vi "pattern_recogn+matching decay.vi"(10 "Image Out":T1, 11 "Path 3":path) -> (1 "Image":T1(plugin-control), 2 "x-y":i32, 3 "Matches (pixel)":T2(array[cluster]))   [LabVIEW 2015]
uses:
  <vilib>/vision/Image Controls.llb/IMAQ Image.ctl
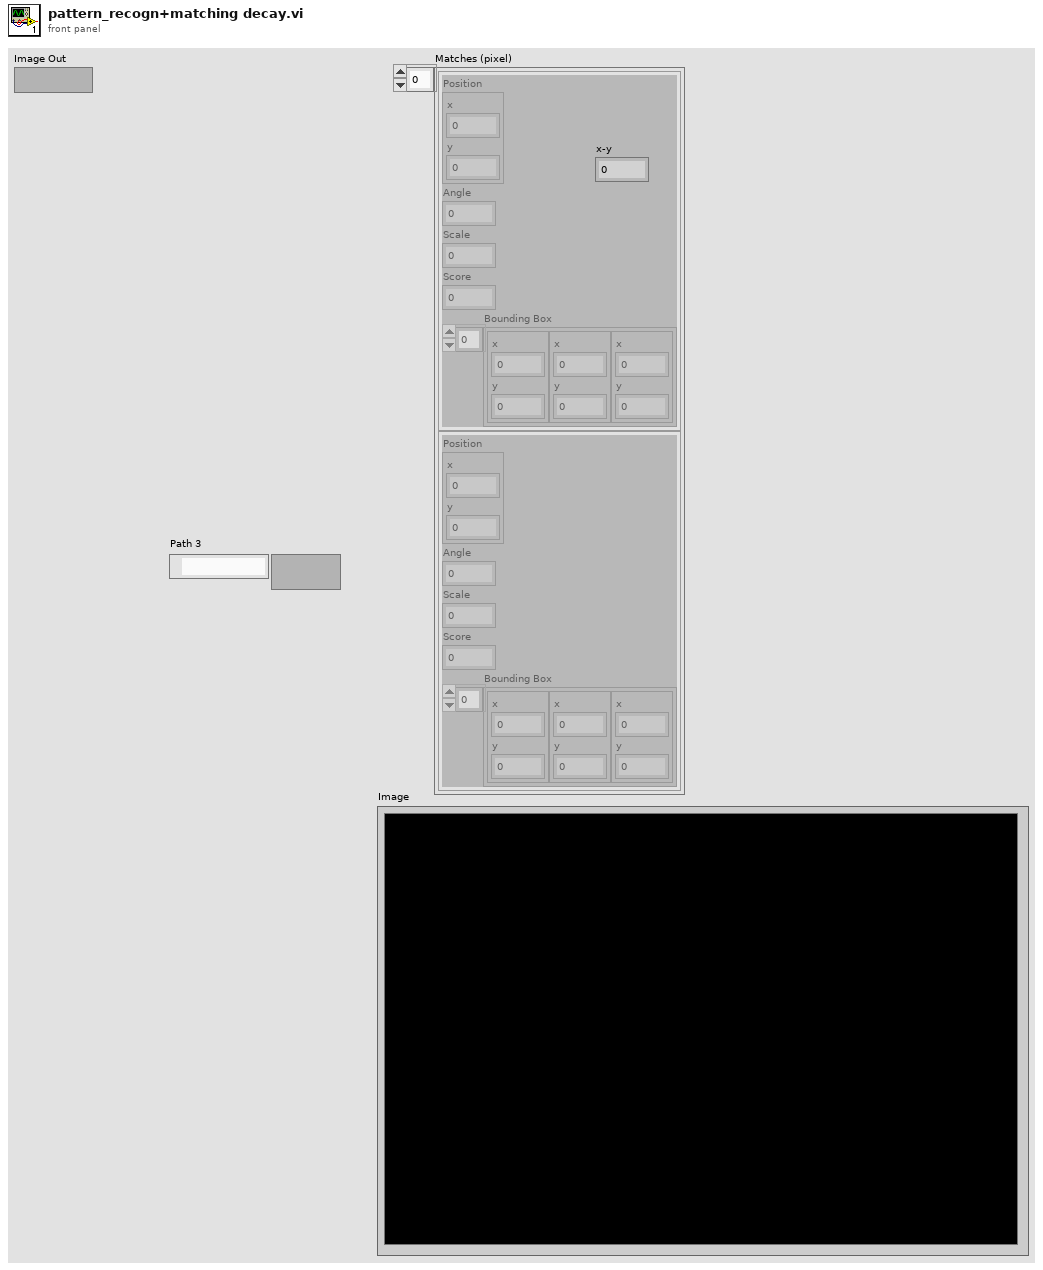
[diagram p1: front panel]
types:
  T1 = typedef "IMAQ Image.ctl" = refnum<image>
  T2 = cluster{"Position":cluster{"x":sgl, "y":sgl}, "Angle":sgl, "Scale":sgl, "Score":sgl, "Bounding Box":cluster{"x":sgl, "y":sgl}[]}[]
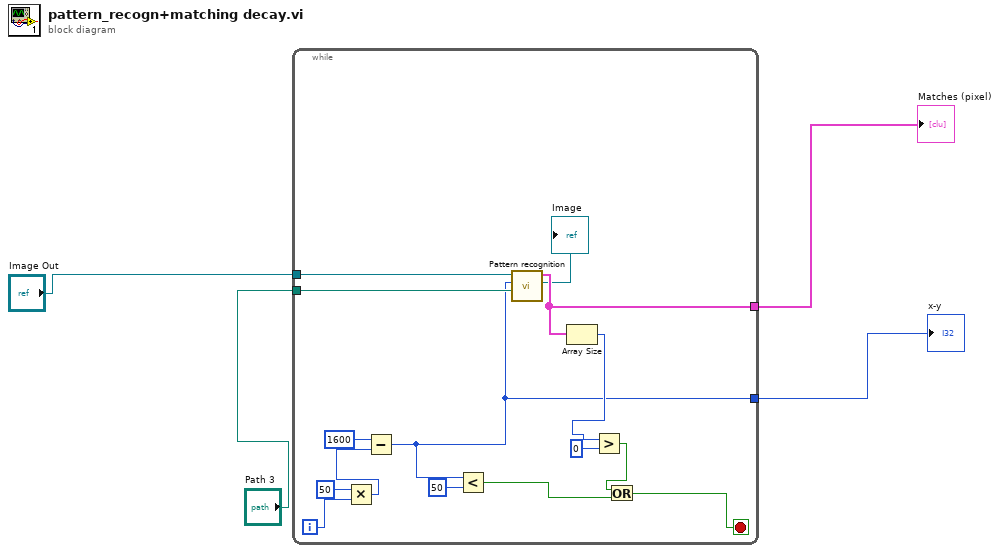
[diagram p0: block diagram]
diagram:
  n1 = while {
    tunnel: "Image Out" -> [w19]
    tunnel: "Path 3" -> [w18]
    tunnel: [w7] -> w2
    tunnel: [w6] -> w3
    i -> [w15]
    stop <- w8 stop-if-true
    n2 = Multiply(x=50, y=w15) -> (x*y=w16:i32)
    n3 = Subtract(x=1600, y=w16) -> (x-y=w6:i32)
    n4 = Less?(x=w6, y=50) -> (x < y?=w9:bool)
    n5 = call "Pattern recognition.vi"("Template Path"=w18, "Minimum match points"=w6, "Image 2"=w19) -> ("Image"=→"Image":T1, "Matches (pixel)"=w7:T2)  [unwired: 7 in]
    n6 = Array Size(array=w7) -> (size(s)=w13:i32)
    n7 = Greater?(x=w13, y=0) -> (0:w10:bool)
    n8 = Or(x=w10, y=w9) -> (x .or. y?=w8:bool)
  }
  "Matches (pixel)" <- w2
  "x-y" <- w3
